vi "send_pause_command.vi"(4 "error in":errorcluster, 7 "Pause":bool) -> (0 "error out":errorcluster)   [LabVIEW 2019, in "Lib_Simx.lvlib"]
doc: "Sends the pause command to server to pause or unpause the update of the ego vehicle on simulation while the simulation keeps going."
uses:
  Lib_Simx.lvlib
  tools/simx_common.vi
panel:
  out "Response":string
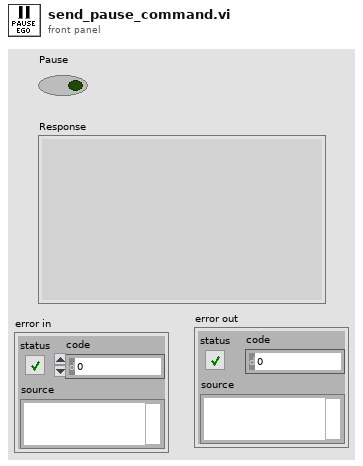
[diagram p1: front panel]
types:
  T1 = typedef "Lib_Simx.lvlib/simx_connection.ctl" = cluster{"Config":T2, "Connections":T5, "Map":cluster{"lanes":cluster{"x":dbl[], "y":dbl[], "z":dbl[]}, "StartPosition":cluster{"start_points":T6, "StartRotation":dbl[], "StartLocation":dbl[]}, "Draw Map Size":T7, "DrawArea":cluster{"min_Y":dbl, "min_X":dbl, "Scale X":dbl, "Scale Y":dbl}, "Map":picture, "Map Geojson":string}}
  T2 = typedef "Lib_Simx.lvlib/config.ctl" = cluster{"Trajectory":T3, "Weather":T4}
  T3 = typedef "Lib_Simx.lvlib/trajectory.ctl" = cluster{"Number of frames":i32, "Frame number":i32, "Trajectory":string}
  T4 = typedef "Lib_Simx.lvlib/weather.ctl" = cluster{"id":string}
  T5 = typedef "Lib_Simx.lvlib/connections.ctl" = cluster{"Simulator Connection":refnum<k5>, "server_ip":string, "Port":i32, "Sensor connections":refnum<k5>[]}
  T6 = typedef "Lib_Simx.lvlib/start_points.ctl" = cluster{"locations":dbl[][], "rotations":dbl[][], "type":string[]}
  T7 = typedef "LVBoundsTypeDef.ctl" = cluster{"Width":u32, "Height":u32}
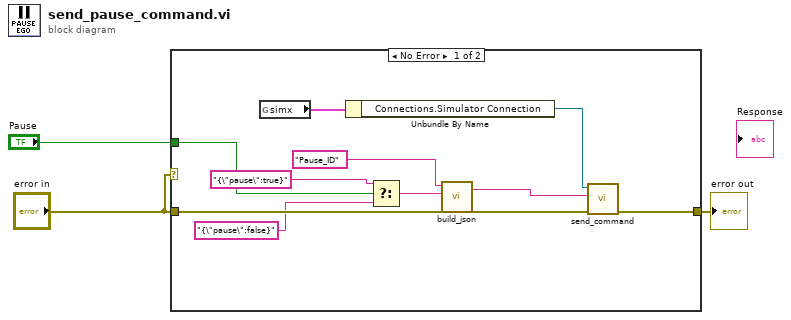
[diagram p0: block diagram]
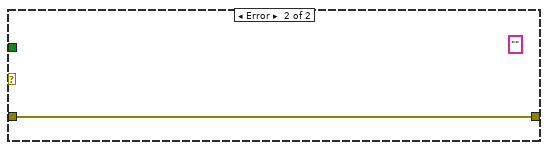
[diagram p2: hidden frame]
diagram:
  n1 = case shown="No Error" "error in" {
    tunnel: "error in" -> [w9 w15]
    tunnel: [w8 w15] -> w2
    tunnel: "Pause" -> [w7 _]
    frame No Error {
      n2 = global read "simx_common.vi" "simx"() -> (w10:T1)
      n3 = Unbundle By Name(w10) -> ("Connections.Simulator Connection"=w13:refnum<k5>)
      n4 = Select(t="{\"pause\":true}" ("Message"), s=w7, f="{\"pause\":false}" ("Message")) -> (s? t:f=w4:string)
      n5 = call "build_json.vi"("error in"=w9, "Message"=w4, "Command_ID"="Pause_ID") -> ("error out"=w14:errorcluster, "JSON Out"=w12:string)  [unwired: 1 in]
      n6 = call "send_command.vi"("error in"=w14, "JSON Command"=w12, "TCP Network Connection in"=w13) -> ("error out"=w8:errorcluster)  [unwired: 1 in, 3 out]
    }
    frame Error {
      (unwired) "" ("Response")
    }
  }
  "error out" <- w2
